vi "队列堆栈（LVObject）.vi"(8 "error in (no error)":errorcluster caption="错误输入（无错误）", 9 "堆栈操作":T1, 10 "堆栈长度":i32=-1, 11 "入栈元素":refnum<class>) -> (0 "error out":errorcluster caption="错误输出", 1 "堆栈空":bool, 3 "出栈元素":refnum<class>)   [LabVIEW 2011]
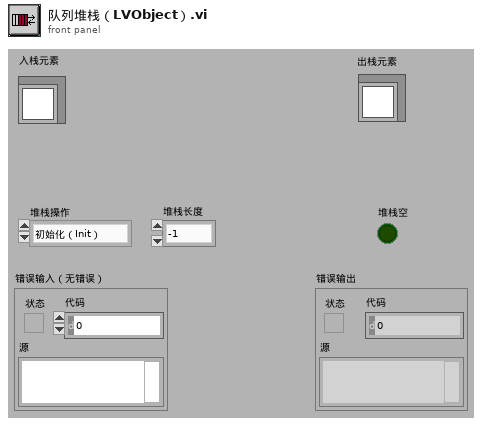
[diagram p1: front panel]
types:
  T1 = typedef "堆栈操作.ctl" = enum16{"初始化（Init）", "进栈（Push）", "出栈（Pop）", "释放"}
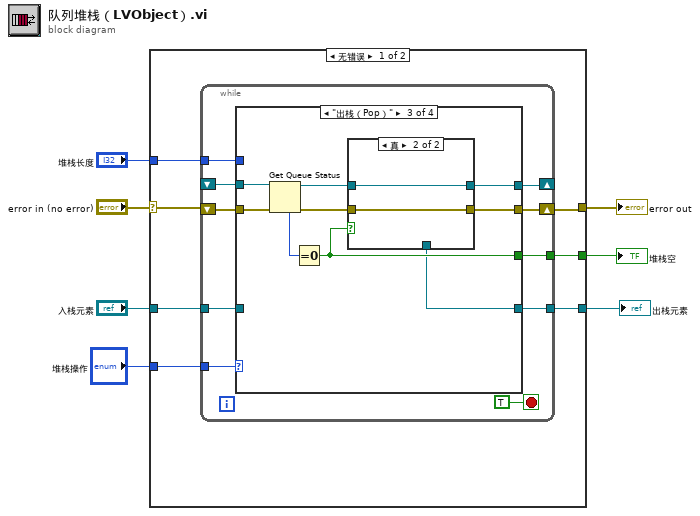
[diagram p0: block diagram]
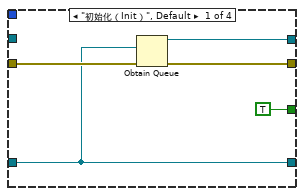
[diagram p2: hidden frame]
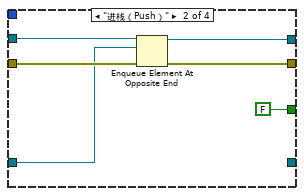
[diagram p3: hidden frame]
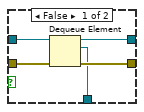
[diagram p4: hidden frame]
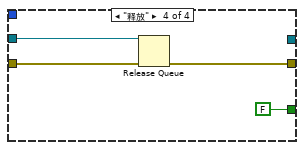
[diagram p5: hidden frame]
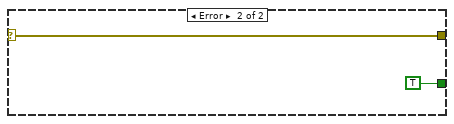
[diagram p6: hidden frame]
diagram:
  n1 = case shown="无错误" "error in (no error)" {
    selector: "error in (no error)" -> [w10 w57]
    tunnel: [w9 w57] -> w6
    tunnel: "堆栈操作" -> [w14 _]
    tunnel: "入栈元素" -> [w13 _]
    tunnel: [w12 _] -> w3
    tunnel: "堆栈长度" -> [w11 _]
    tunnel: [w8 TRUE] -> w1
    frame No Error {
      n2 = while {
        tunnel: w14 -> [w24]
        tunnel: w13 -> [w23]
        tunnel: [w22] -> w12
        tunnel: w11 -> [w21]
        shift-right: [w18] -> w9
        shift-left: w10 -> [w19]
        shift-right: [w17] -> _
        shift-left: _ -> [w16]
        tunnel: [w15] -> w8
        stop <- TRUE stop-if-true
        n3 = case shown="\"出栈（Pop）\"" w24 {
          tunnel: w23 -> [w26 w31 _ _]
          tunnel: [w26 _ w36 _] -> w22
          tunnel: w21 -> [_ _ _ _]
          tunnel: w19 -> [w29 w35 w44 w55]
          tunnel: [w28 w34 w37 w54] -> w18
          tunnel: [w27 w32 w39 _] -> w17
          tunnel: w16 -> [_ w33 w43 w53]
          tunnel: [TRUE FALSE w41 FALSE] -> w15
          frame "初始化（Init）", Default {
            n4 = Obtain Queue(element data type=w26, error in (no error)=w29) -> (queue out=w27:refnum<queue>, error out=w28:errorcluster)  [unwired: 3 in, 1 out]
          }
          frame "进栈（Push）" {
            n5 = Enqueue Element At Opposite End(queue=w33, element=w31, error in (no error)=w35) -> (queue out=w32:refnum<queue>, error out=w34:errorcluster)  [unwired: 1 in, 1 out]
          }
          frame "出栈（Pop）" {
            n6 = Get Queue Status(queue=w43, error in (no error)=w44) -> (queue out=w40:refnum<queue>, error out=w38:errorcluster, # elements in queue=w42:i32)  [unwired: 1 in, 5 out]
            n7 = Equal To 0?(x=w42) -> (x = 0?=w41:bool)
            n8 = case shown="真" w41 {
              tunnel: w40 -> [w49 w51]
              tunnel: [w48 w51] -> w39
              tunnel: w38 -> [w47 w50]
              tunnel: [w46 w50] -> w37
              tunnel: [w45 _] -> w36
              frame False {
                n9 = Dequeue Element(queue=w49, error in (no error)=w47) -> (queue out=w48:refnum<queue>, element=w45:refnum<class>, error out=w46:errorcluster)  [unwired: 1 in, 1 out]
              }
              frame True {
              }
            }
          }
          frame "释放" {
            n10 = Release Queue(queue=w53, error in (no error)=w55) -> (error out=w54:errorcluster)  [unwired: 1 in, 2 out]
          }
        }
      }
    }
    frame Error {
    }
  }
  "error out" <- w6
  "出栈元素" <- w3
  "堆栈空" <- w1
